vi "Dequeue_Elements.vi"(4 "error in (no error)":errorcluster, 7 "Queue in":refnum<queue>) -> (0 "error out":errorcluster, 1 "Data":variant, 2 "State":T1, 3 "queue out":refnum<queue>)   [LabVIEW 2023]
doc: "Get the data from the queue"
uses:
  Controls/State.ctl
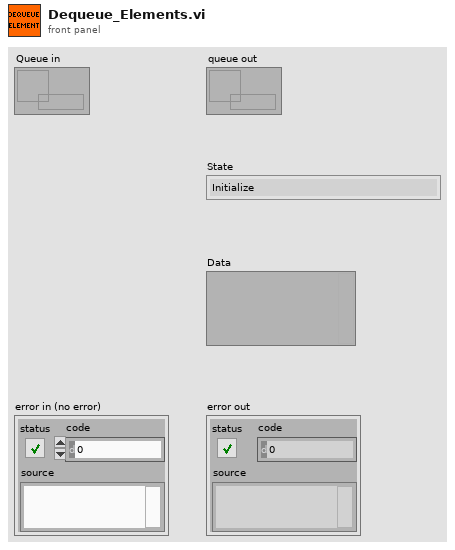
[diagram p1: front panel]
types:
  T1 = typedef "State.ctl" = enum16{"Initialize", "Wait for Something", "Step Completed", "Save Wash Options", "Start Process", "Car Position", "Order Steps to follow", "Underbody Wash", "Bug Remover", "Pre-Soak", "High Pressure Wash", "Low Pressure Wax", "Spot Free Rinse", "Tire Shine Foam", "Air Dry", "Vehicle out of position", "Exit", "Process Complete", "Stop Application"}
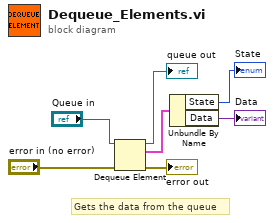
[diagram p0: block diagram]
diagram:
  # "Gets the data from the queue"
  n1 = Dequeue Element(queue="Queue in", error in (no error)="error in (no error)") -> (queue out=→"queue out":refnum<queue>, element=w5:cluster{"State":T1, "Data":variant}, error out=→"error out":errorcluster)  [unwired: 1 in, 1 out]
  n2 = Unbundle By Name(w5) -> ("State"=→"State":T1, "Data"=→"Data":variant)
